vi "Wybór z tablicy SubVI.vi"(8 "error in":errorcluster, 10 "Numeric":u16) -> (0 "error out":errorcluster, 2 "Enum":T1)   [LabVIEW 2015]
uses:
  Controls/States.ctl
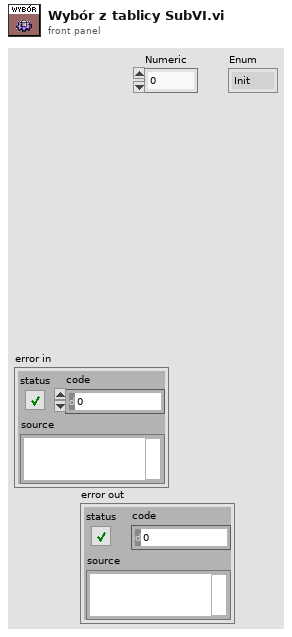
[diagram p1: front panel]
types:
  T1 = typedef "States.ctl" = enum16{"Init", "Idle", "Cotton", "Silk", "Fast", "Drying"}
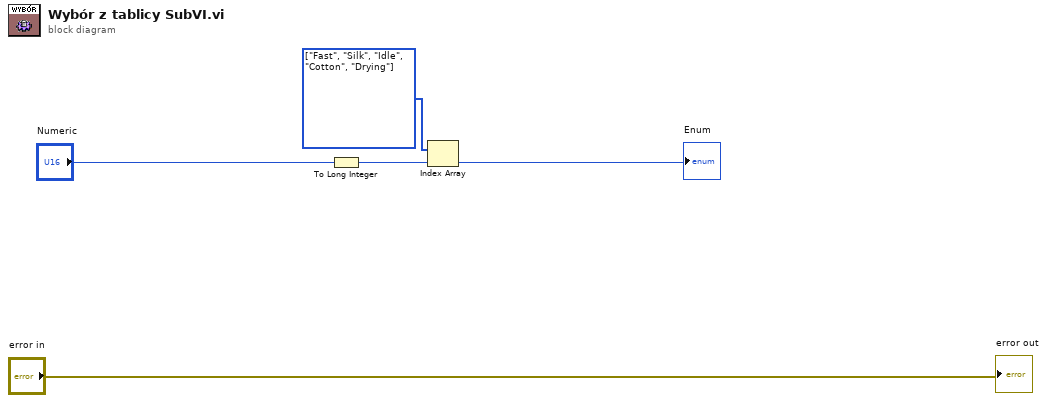
[diagram p0: block diagram]
diagram:
  w2 = T1[] [enum."Fast", enum."Silk", enum."Idle", enum."Cotton", enum."Drying"] items=["Init", "Idle", "Cotton", "Silk", "Fast", "Drying"]
  n1 = To Long Integer(number="Numeric") -> (32bit integer=w3:i32)
  n2 = Index Array(array=w2, index=w3) -> (element=→"Enum":T1)
  "error out" <- "error in"
